vi "Generate CSV Report.vi"(0 "Serial Number":string, 1 "Date":string, 2 "Test Number":string[](array[string]), 3 "Time":string, 4 "Retest":string, 5 "Lower Limits":dbl[](array[numeric]), 6 "Measurment values":dbl[](array[numeric]), 8 "Fixture":string, 9 "Upper Limits":dbl[](array[numeric]), 12 "Variant":string, 13 "Status":string[](array[string]), 14 "Project":string, 15 "Overall status":string, 17 "Test Names":string[](array[string])) -> (27 "error out":errorcluster)   [LabVIEW 2023, in "CSV Report.lvlib"]
uses:
  CSV Report.lvlib
  <vilib>/Utility/file.llb/Write Delimited Spreadsheet (string).vi
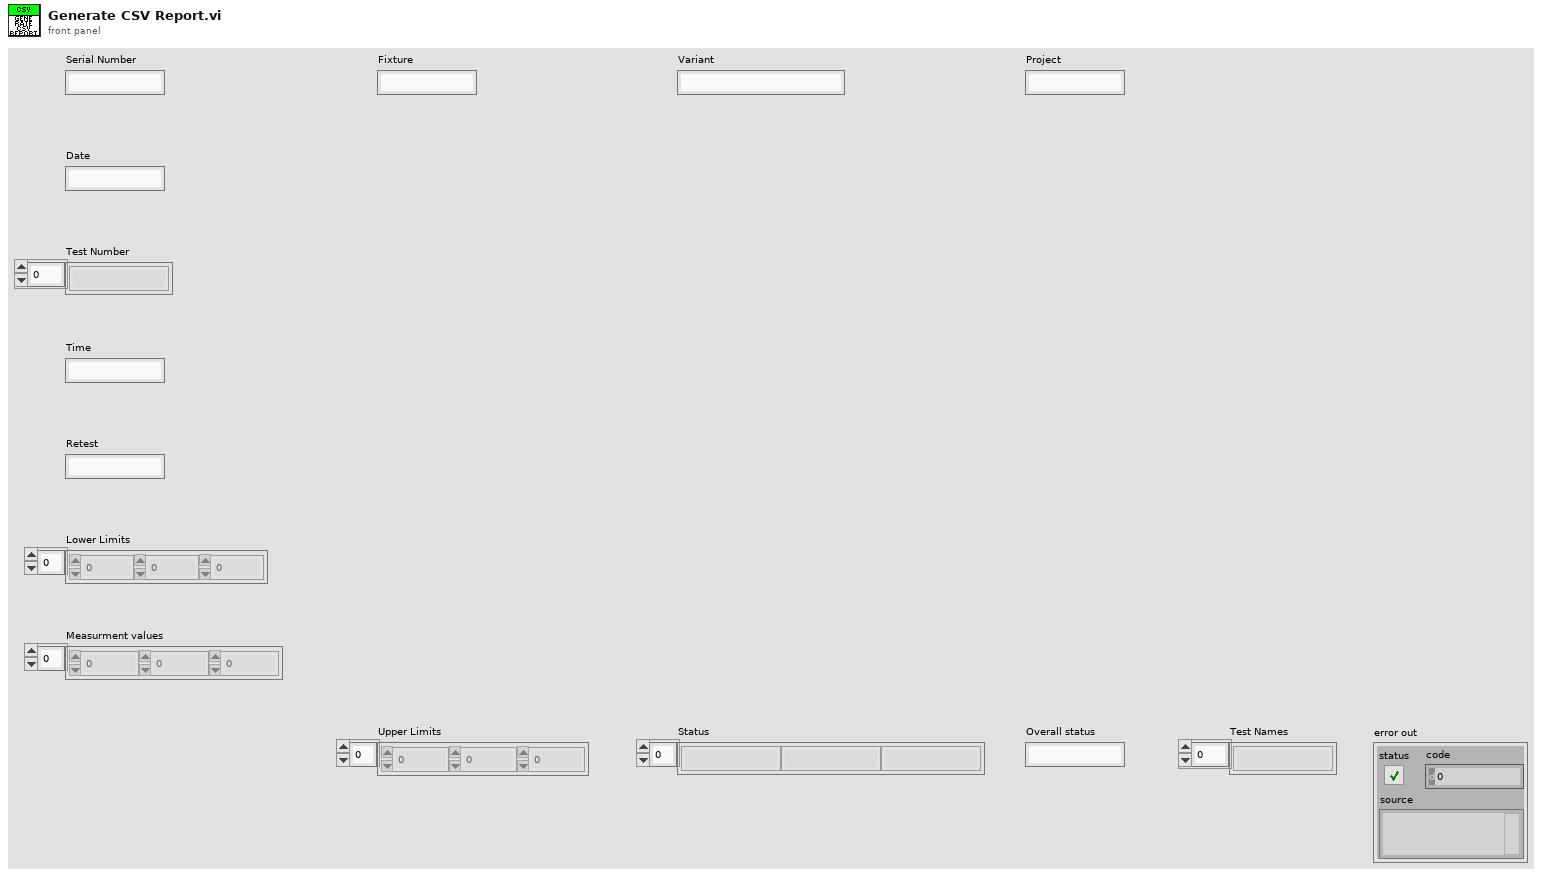
[diagram p1: front panel]
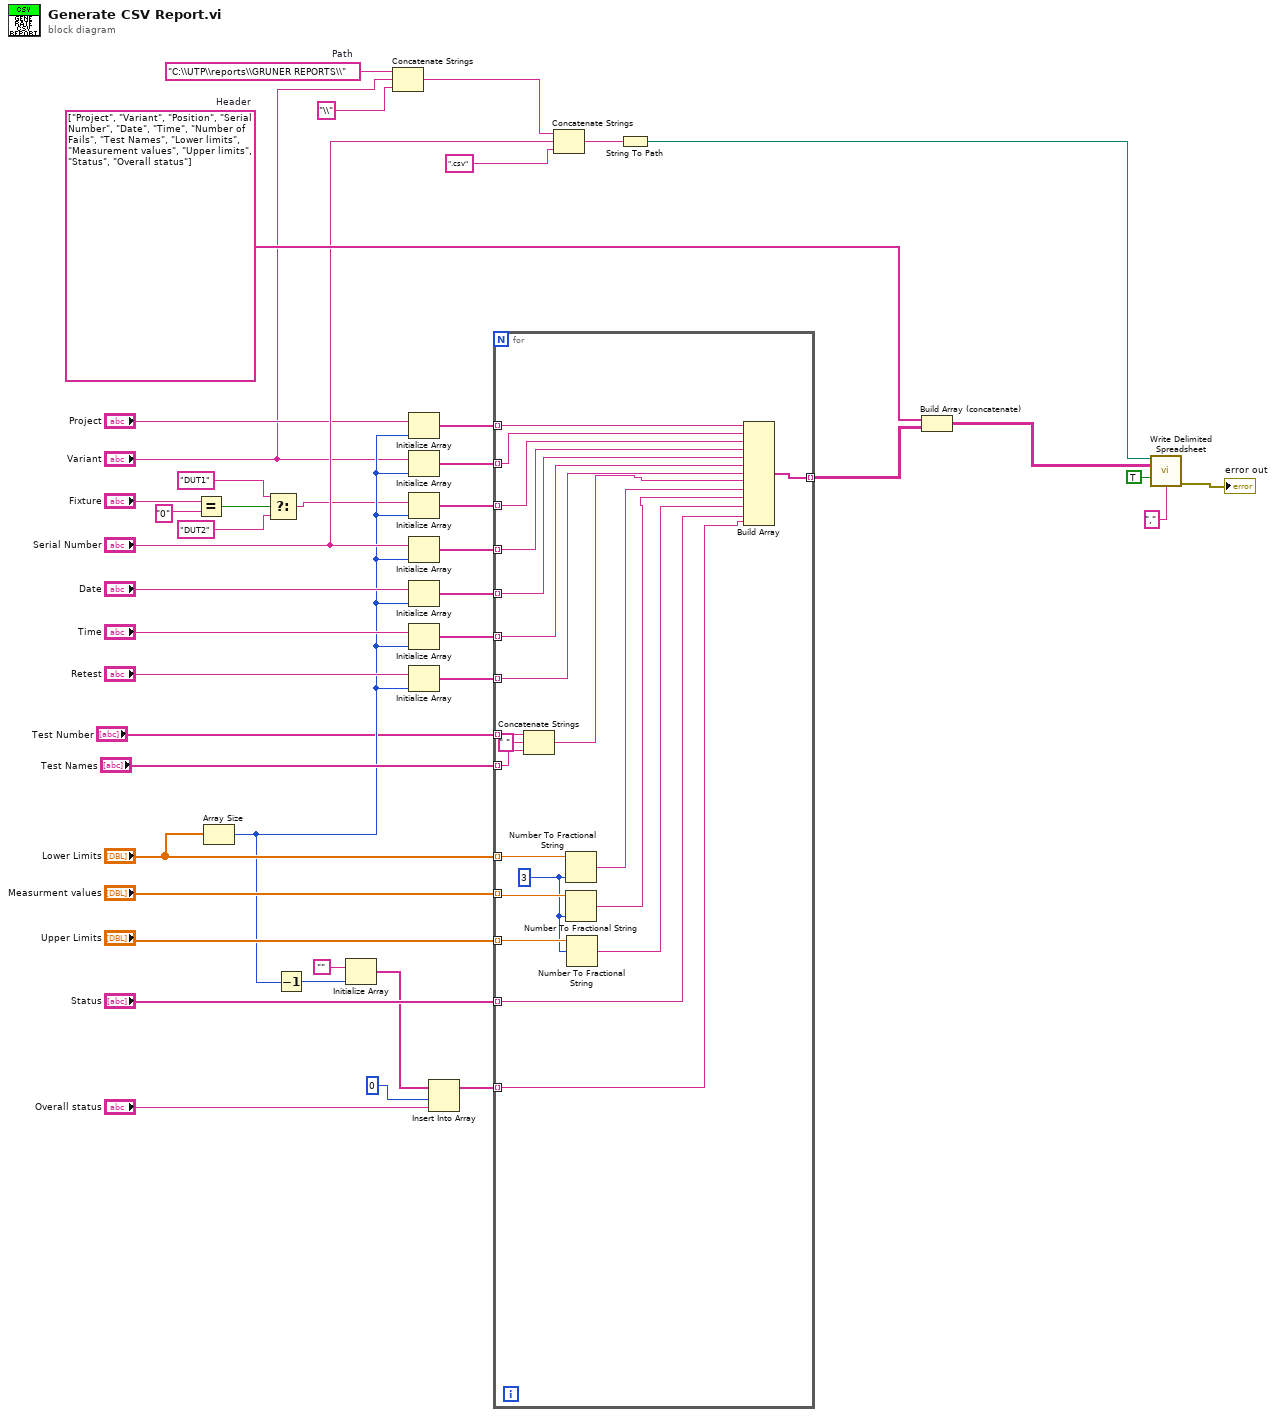
[diagram p0: block diagram]
diagram:
  w11 = "C:\\UTP\\reports\\GRUNER REPORTS\\"  # Path
  w32 = string[] ["Project", "Variant", "Position", "Serial Number", "Date", "Time", "Number of Fails", "Test Names", "Lower limits", "Measurement values", "Upper limits", "Status", "Overall status"]  # Header
  n1 = Equal?(x="Fixture", y="0") -> (x = y?=w4:bool)
  n2 = Array Size(array="Lower Limits") -> (size(s)=w13:i32)
  n3 = Select(t="DUT1" ("y"), s=w4, f="DUT2" ("y")) -> (s? t:f=w1:string)
  n4 = Decrement(x=w13) -> (x-1=w22:i32)
  n5 = Initialize Array("", w22) -> (w15:string[])
  n6 = Concatenate Strings(w11, "Variant", "\\" ("string")) -> (w8:string)
  n7 = Initialize Array("Project", w13) -> (w44:string[])
  n8 = Initialize Array("Variant", w13) -> (w43:string[])
  n9 = Initialize Array(w1, w13) -> (w42:string[])
  n10 = Initialize Array("Serial Number", w13) -> (w33:string[])
  n11 = Initialize Array("Date", w13) -> (w41:string[])
  n12 = Initialize Array("Time", w13) -> (w40:string[])
  n13 = Initialize Array("Retest", w13) -> (w29:string[])
  n14 = Insert Into Array(array=w15, index=0, new element="Overall status") -> (w35:string[])
  n15 = for {
    tunnel: w44 -> [w60] mode=indexing
    tunnel: w43 -> [w59] mode=indexing
    tunnel: w42 -> [w58] mode=indexing
    tunnel: w33 -> [w57] mode=indexing
    tunnel: w41 -> [w56] mode=indexing
    tunnel: w40 -> [w55] mode=indexing
    tunnel: "Lower Limits" -> [w65] mode=indexing
    tunnel: "Measurment values" -> [w64] mode=indexing
    tunnel: "Upper Limits" -> [w63] mode=indexing
    tunnel: "Status" -> [w48] mode=indexing
    tunnel: w35 -> [w47] mode=indexing
    tunnel: [w61] -> w31 mode=indexing
    tunnel: w29 -> [w54] mode=indexing
    tunnel: "Test Names" -> [w46] mode=indexing
    tunnel: "Test Number" -> [w53] mode=indexing
    w62 = i16 3 ("precision (6)")
    n16 = Concatenate Strings(w53, " " ("string"), w46) -> (w52:string)
    n17 = Number To Fractional String(number=w65, precision (6)=w62) -> (F-format string=w51:string)  [unwired: 2 in]
    n18 = Number To Fractional String(number=w64, precision (6)=w62) -> (F-format string=w50:string)  [unwired: 2 in]
    n19 = Number To Fractional String(number=w63, width (-)=w62) -> (F-format string=w49:string)  [unwired: 2 in]
    n20 = Build Array(w60, w59, w58, w57, w56, w55, w54, w52, w51, w50, w49, w48, w47) -> (w61:string[])
  }
  n21 = Concatenate Strings(w8, "Serial Number", ".csv" ("string")) -> (w28:string)
  n22 = String To Path(string=w28) -> (path=w27:path)
  n23 = Build Array (concatenate)(w32, w31) -> (w30:string[][])
  n24 = call-poly <vilib>:"Write Delimited Spreadsheet.vi"("file path (dialog if empty)"=w27, "2D data"=w30, "append to file? (new file:F)"=TRUE, "delimiter (\\t)"="," ("delimiter (\\t)")) -> ("error out"=→"error out":errorcluster)  [unwired: 10 in, 1 out]
